vi "subRetrieveAccelValues.vi"(2 "error in":errorcluster, 3 "AccelState":refnum<k24>, 4 "WiimoteState":refnum<k24>) -> (0 "error out":errorcluster, 1 "Wiimote State":T1)   [LabVIEW 2010]
uses:
  C:/Users/×ñÞóôïò/Desktop/rtdsp_project14_4_11/3D_Experiment/libs/ola/WiimoteManaged(wml17)/WiimoteLib.dll
  WiimoteLib.dll
  wiimotestate.ctl
panel:
  # "Accelerometers"
  # "Buttons"
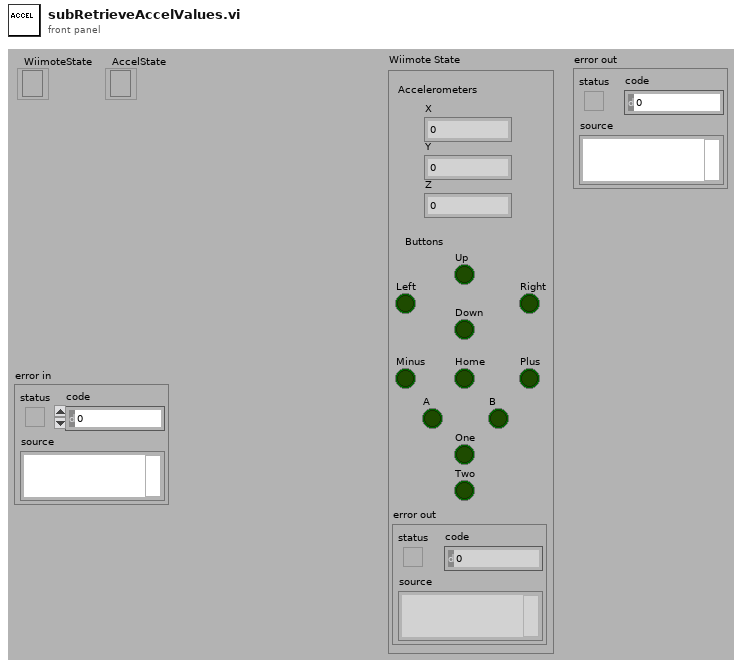
[diagram p1: front panel]
types:
  T1 = typedef "wiimotestate.ctl" = cluster{"X":sgl, "Y":sgl, "Z":sgl, "A":bool, "B":bool, "Down":bool, "Home":bool, "Left":bool, "Minus":bool, "One":bool, "Plus":bool, "Right":bool, "Two":bool, "Up":bool, "error out":errorcluster}
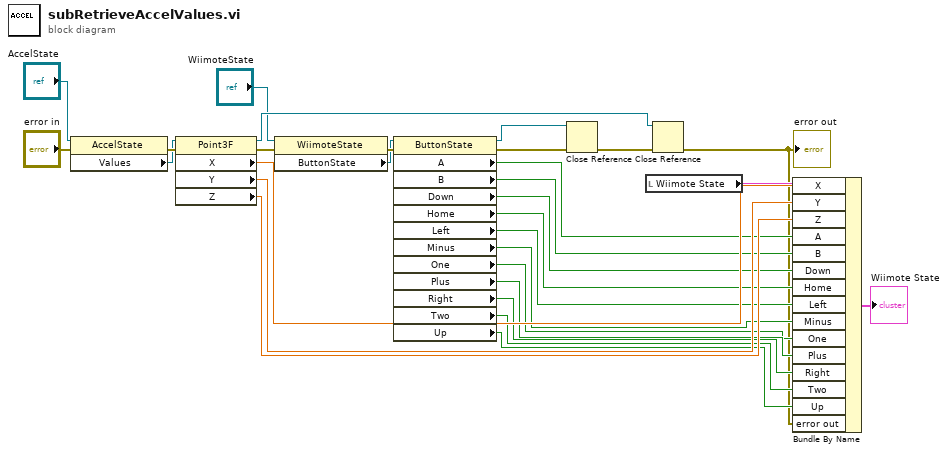
[diagram p0: block diagram]
diagram:
  n1 = property class="AccelState"(reference="AccelState", error in="error in") -> (error out=w25:errorcluster, "Values"=w17:refnum<k24>)  [unwired: 1 out]
  n2 = property class="Point3F"(reference=w17, error in=w25) -> (reference out=w26:refnum<k24>, error out=w29:errorcluster, "X"=w18:sgl, "Y"=w19:sgl, "Z"=w20:sgl)
  n3 = property class="WiimoteState"(reference="WiimoteState", error in=w29) -> (error out=w23:errorcluster, "ButtonState"=w22:refnum<k24>)  [unwired: 1 out]
  n4 = property class="ButtonState"(reference=w22, error in=w23) -> (reference out=w24:refnum<k24>, error out=w27:errorcluster, "A"=w5:bool, "B"=w6:bool, "Down"=w7:bool, "Home"=w8:bool, "Left"=w9:bool, "Minus"=w10:bool, "One"=w11:bool, "Plus"=w12:bool, "Right"=w13:bool, "Two"=w14:bool, "Up"=w15:bool)
  n5 = Close Reference(reference=w24, error in (no error)=w27) -> (error out=w1:errorcluster)
  n6 = local read "Wiimote State"() -> (w3:T1)
  n7 = Close Reference(reference=w26, error in (no error)=w1) -> (error out=w2:errorcluster)
  "error out" <- w2
  n8 = Bundle By Name(cluster=w3, "X"=w18, "Y"=w19, "Z"=w20, "A"=w5, "B"=w6, "Down"=w7, "Home"=w8, "Left"=w9, "Minus"=w10, "One"=w11, "Plus"=w12, "Right"=w13, "Two"=w14, "Up"=w15, "error out"=w2) -> (→"Wiimote State":T1)
